vi "Stage v3.vi"() -> ()   [LabVIEW 2025]
uses:
  upper limit.ctl
  lower limit.ctl
  libximc.lvlib
panel:
  in  "Help":bool
  in  "Shift Stage Page":bool
  in  "Move to Destination Page":bool
  in  "Move Relative Page":bool
  in  "Initialize Page":bool
  in  "Tab Control":T1(tab)=enum."Shift Stage"
  out "s/n 2":u32
  out "s/n 3":u32
  out "s/n 1":u32
  in  "Controller 1":u16(ring) items=["xi-com:\\\\.\\COM4", "xi-com:\\\\.\\COM5", "xi-com:\\\\.\\COM6"]
  in  "Controller 2":u16(ring) items=["xi-com:\\\\.\\COM4", "xi-com:\\\\.\\COM5", "xi-com:\\\\.\\COM6"]
  in  "Controller 3":u16(ring) items=["xi-com:\\\\.\\COM4", "xi-com:\\\\.\\COM5", "xi-com:\\\\.\\COM6"]
  in  "Move To Destination":bool
  in  "Destination X":i32
  in  "Destination Z":i32
  in  "Destination Y":i32
  in  "Update Position":bool
  in  "Paste Positions":bool
  in  "Shift X":i32
  in  "Shift Z":i32
  in  "Shift Y":i32
  in  "Move Relative":bool
  in  "shift stage":bool
  in  "Shift Amount (Steps)":i32
  in  "Copy Positions":bool
  out "/256":i32
  out "/256":i32
  out "/256":i32
  in  "Zero":bool
  in  "Go Home":bool
  in  "Exit":bool
  out "Cursor X":dbl format="%#.2f"
  out "Cursor Z":dbl format="%#.2f"
  out "Cursor Y":dbl format="%#.2f"
  # "Controller IDs"
  # "Serial Numbers"
  # "Controller X"
  # "Controller Y"
  # "Controller Z"
  # "If serial numbers are 0, click the help button!"
  # "NOTE: Units of all positions are in steps."
  # "Stage not moving:"
  # "Check if the serial numbers are zero. If so, close this app and load the controllers in order (1, 2, then 3) in XILab. Close XILab and open this app. and controllers should load correctly."
  # "Controllers not found in XILab:"
  # "Unplug and replug USBs connecting the motors to the computer, then follow previous instructions."
  # "If you have any other questions, feel free to reach out to Erykah at erykahfoss@u.boisestate.edu"
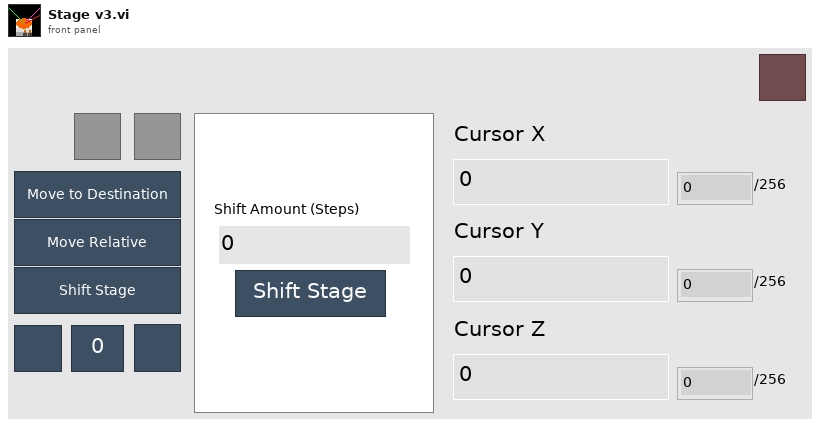
[diagram p1: front panel]
types:
  T1 = enum32{"Initialize", "Help", "Move to Destination", "Move Relative", "Shift Stage"}
  T2 = enum16{"Initialize", "Help", "Move to Destination", "Move Relative", "Shift Stage"}
  T3 = enum32{"invalid app kind", "Development System", "Run Time System", "Student Edition", "Embedded LabVIEW", "Evaluation", "Custom"}
  T4 = cluster{"Number of controllers":i32, "Controllers' names":string[], "variant":variant, "quit":bool, "IDs":i32[]}
  T5 = typedef "eventvkey.ctl" = enum16{"ASCII", "Enter", "Return", "Shift", "Ctrl", "Alt", "Cmd", "Opt", "Caps", "NumLock", "Clear", "Break", "Up", "Down", "Left", "Right", "Insert", "Delete", "Home", "End", "PageUp", "PageDown", "Escape", "Help", "Pause", "ScrollLock", "F1", "F2", "F3", "F4", "F5", "F6", "F7", "F8", "F9", "F10", "F11", "F12", "F13", "F14", "F15", "F16", "F17", "F18", "F19", "F20", "F21", "F22", "F23", "F24", "Play", "VolumeUp", "VolumeDown", "Mute", "Two Byte Char"}
  T6 = typedef "lower limit.ctl" = i32
  T7 = typedef "upper limit.ctl" = i32
  T8 = cluster{"MoveSts":u32, "MvCmdSts":u32, "PWRSts":u32, "EncSts":u32, "WindSts":u32, "CurPosition":i32, "uCurPosition":i32, "@dummy control@":i8, "@dummy control@":i8, "@dummy control@":i8, "@dummy control@":i8, "EncPosition":i64, "CurSpeed":i32, "uCurSpeed":i32, "Ipwr":i32, "Upwr":i32, "Iusb":i32, "Uusb":i32, "CurT":i32, "Flags":u32, "GPIOFlags":u32, "CmdBufFreeSpace":u32}
  T9 = cluster{"Shift Y":i32, "Shift Z":i32, "Shift X":i32}
  T10 = cluster{"Destination Y":i32, "Destination Z":i32, "Destination X":i32}
  T11 = cluster{"Shift Amount (Steps)":i32, "Shift Amount (Steps)":i32, "Shift Amount (Steps)":i32}
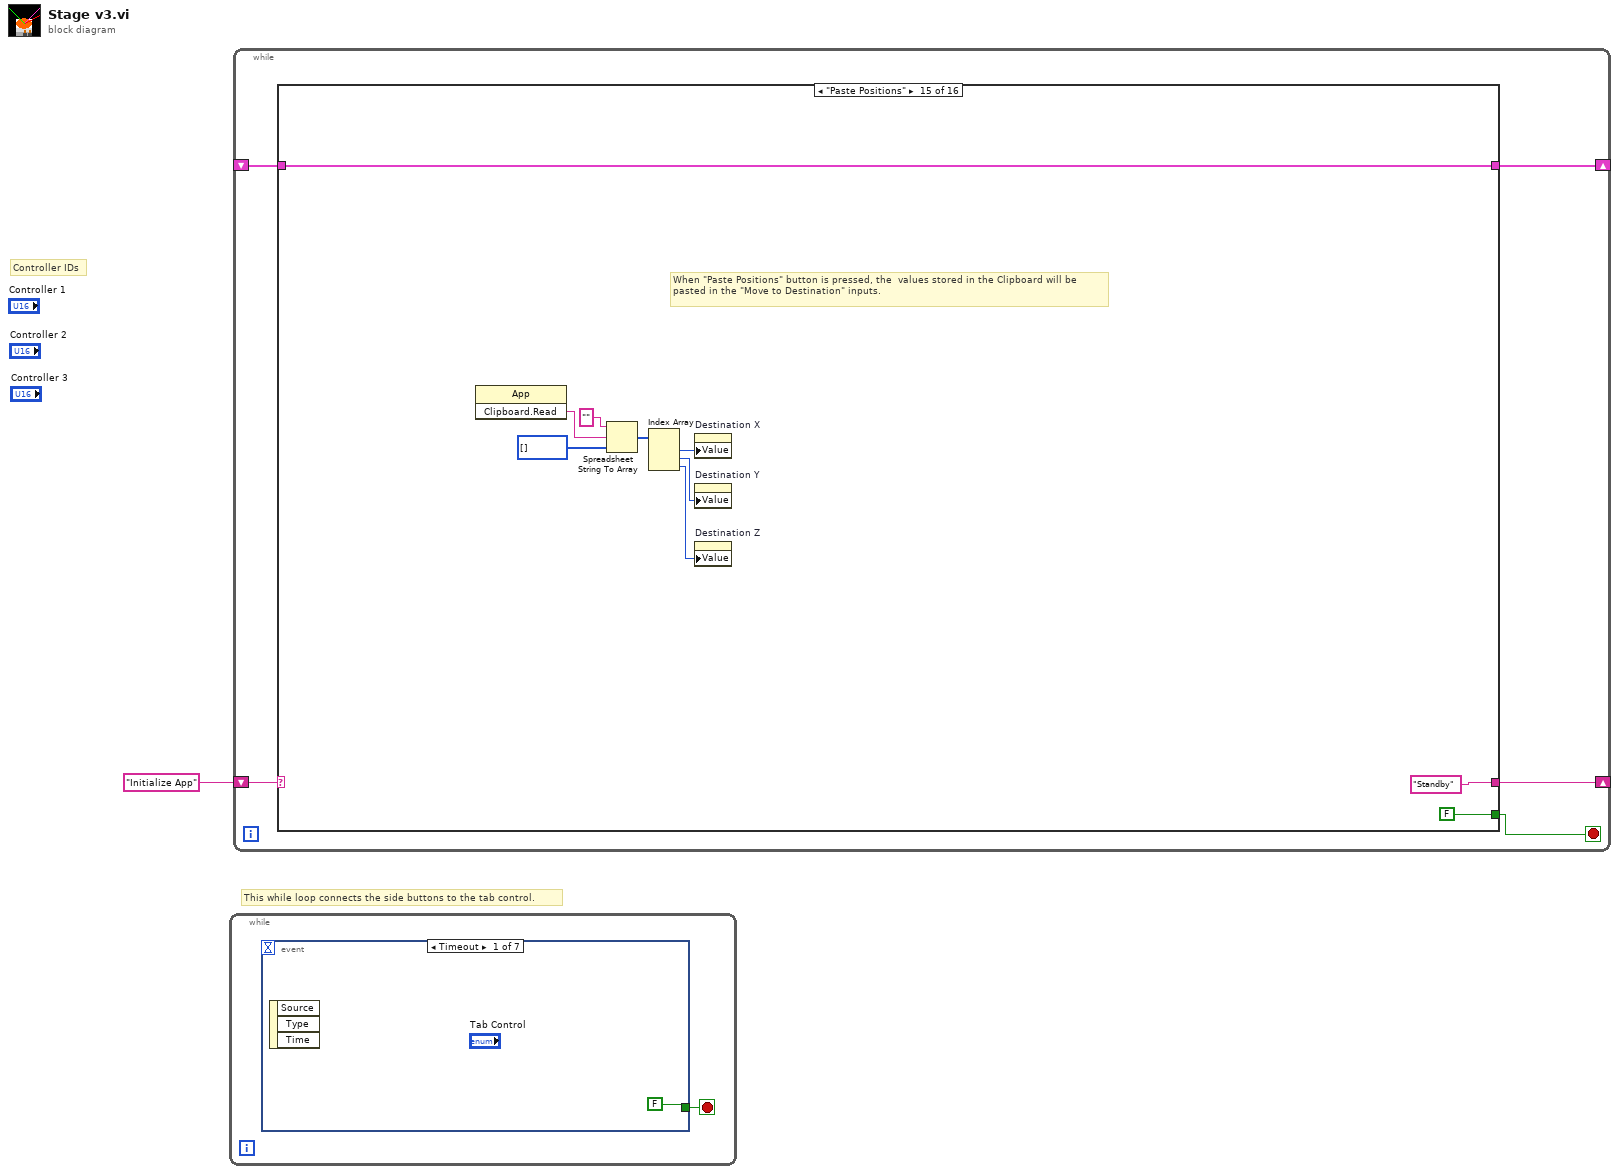
[diagram p0: block diagram]
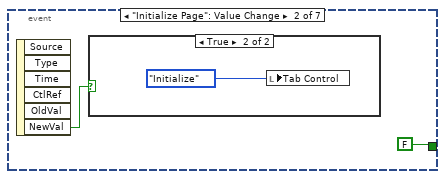
[diagram p2: hidden frame]
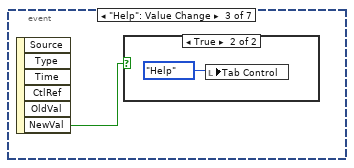
[diagram p4: hidden frame]
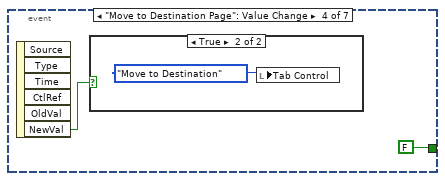
[diagram p6: hidden frame]
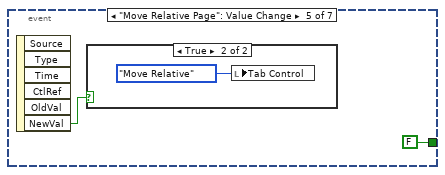
[diagram p8: hidden frame]
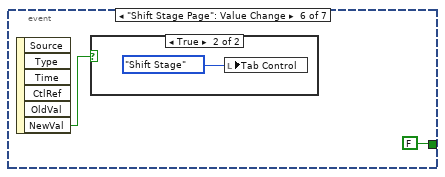
[diagram p10: hidden frame]
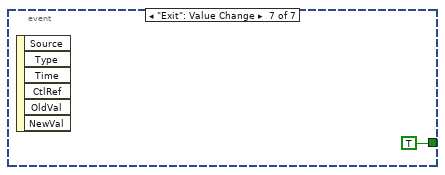
[diagram p12: hidden frame]
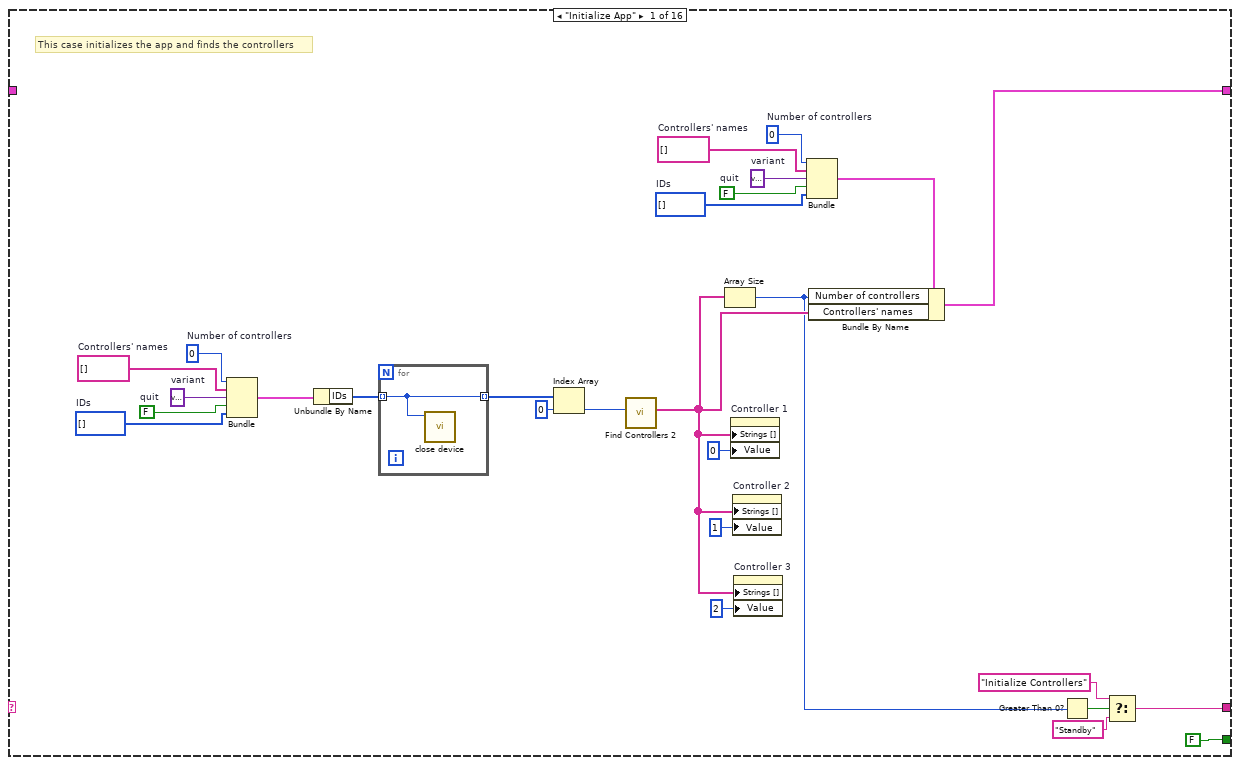
[diagram p13: hidden frame]
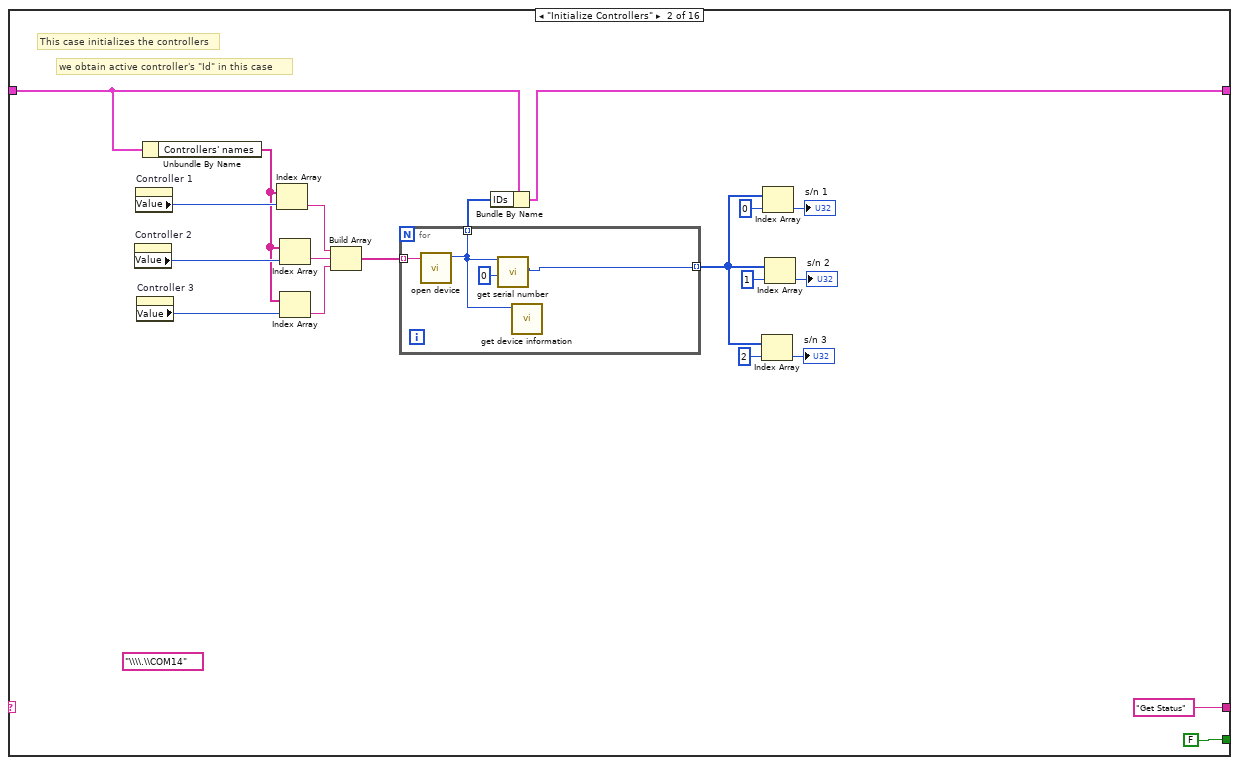
[diagram p14: hidden frame]
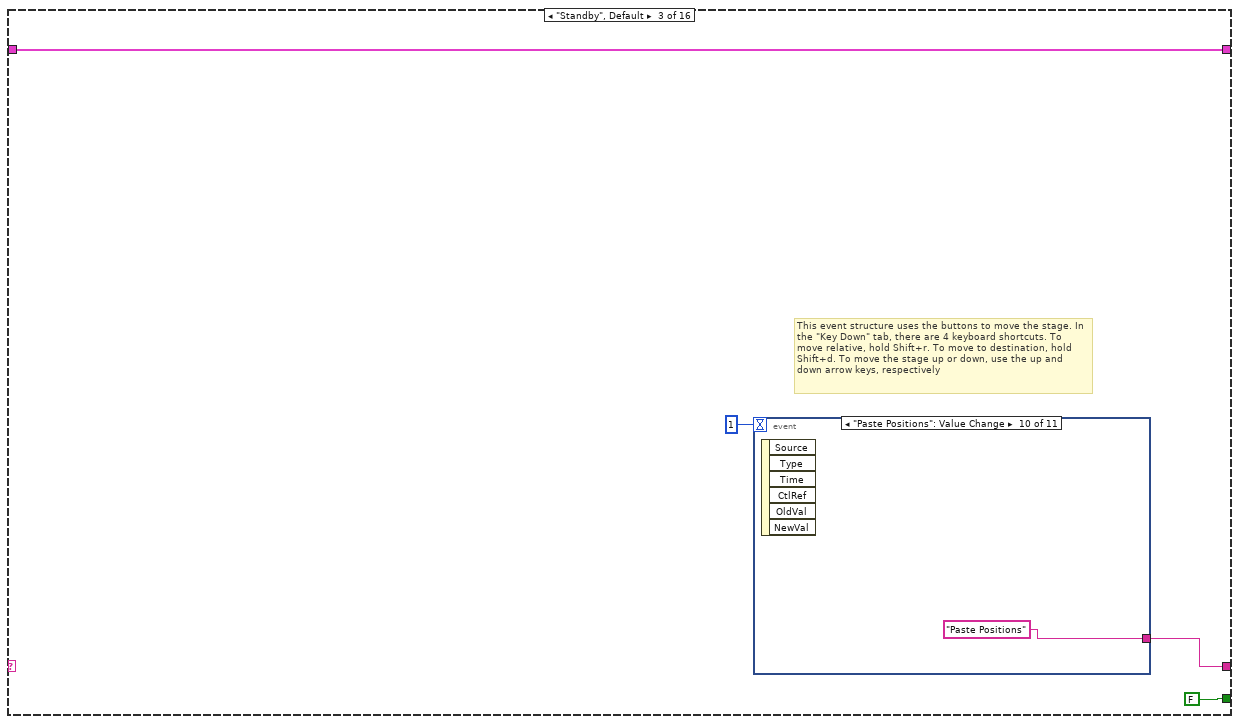
[diagram p15: hidden frame]
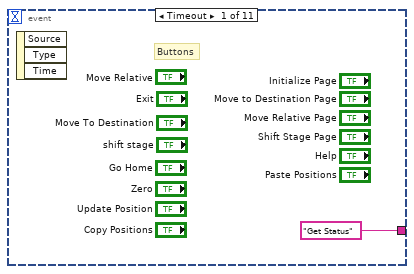
[diagram p16: hidden frame]
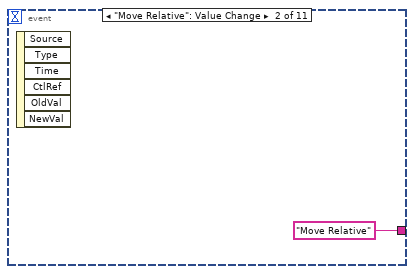
[diagram p17: hidden frame]
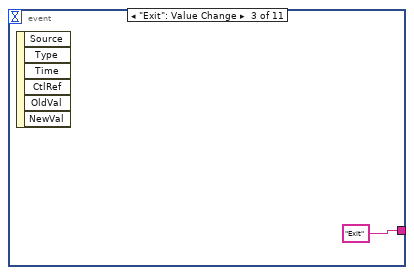
[diagram p18: hidden frame]
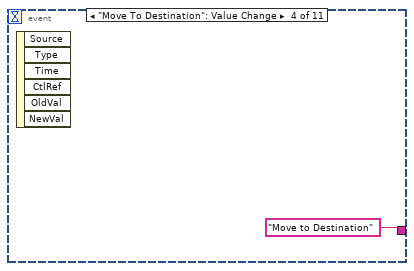
[diagram p19: hidden frame]
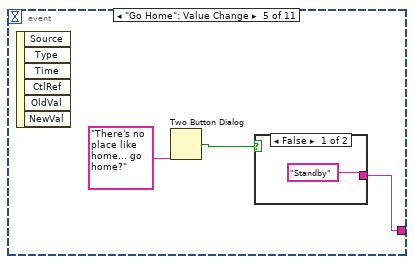
[diagram p20: hidden frame]
diagram:
  # "This while loop connects the side buttons to the tab control."
  # "Controller IDs"
  n1 = while {
    stop <- w2 stop-if-true
    n2 = event shown="[0] Timeout" {
      selector: _ -> [_ _ _ _ _ _ _]
      dyn-events: _ -> [_ _ _ _ _ _ _]
      timeout: _ -> [_ _ _ _ _ _ _]
      tunnel: [FALSE FALSE _ FALSE FALSE FALSE TRUE] -> w2
      event Timeout {
        n3 = event-data() -> ()  [unwired: 1 in, 3 out]
      }
      event "Initialize Page": Value Change {
        n4 = event-data() -> ("NewVal"=w4:bool)  [unwired: 1 in, 5 out]
        n5 = case shown="True" w4 {
          frame False {
          }
          frame True {
            n6 = local write "Tab Control"(T2."Initialize") -> ()
          }
        }
      }
      event "Help": Value Change {
        n7 = event-data() -> ("NewVal"=w7:bool)  [unwired: 1 in, 5 out]
        n8 = case shown="True" w7 {
          frame False {
          }
          frame True {
            n9 = local write "Tab Control"(T2."Help") -> ()
          }
        }
      }
      event "Move to Destination Page": Value Change {
        n10 = event-data() -> ("NewVal"=w9:bool)  [unwired: 1 in, 5 out]
        n11 = case shown="True" w9 {
          frame False {
          }
          frame True {
            n12 = local write "Tab Control"(T2."Move to Destination") -> ()
          }
        }
      }
      event "Move Relative Page": Value Change {
        n13 = event-data() -> ("NewVal"=w12:bool)  [unwired: 1 in, 5 out]
        n14 = case shown="True" w12 {
          frame False {
          }
          frame True {
            n15 = local write "Tab Control"(T2."Move Relative") -> ()
          }
        }
      }
      event "Shift Stage Page": Value Change {
        n16 = event-data() -> ("NewVal"=w15:bool)  [unwired: 1 in, 5 out]
        n17 = case shown="True" w15 {
          frame False {
          }
          frame True {
            n18 = local write "Tab Control"(T2."Shift Stage") -> ()
          }
        }
      }
      event "Exit": Value Change {
        n19 = event-data() -> ()  [unwired: 1 in, 6 out]
      }
    }
  }
  n20 = while {
    shift-right: [w22] -> _
    shift-left: _ -> [w23]
    shift-right: [w21] -> _
    shift-left: "Initialize App" -> [w20]
    stop <- w19 stop-if-true
    n21 = case shown="\"Paste Positions\"" w20 {
      tunnel: [w44 w61 w79 w118 w175 w236 w284 w341 w400 w449 w454 w459 w467 w489 w499 w507] -> w22
      tunnel: w23 -> [_ w62 w79 w118 w175 w235 w284 w341 w400 w449 w454 w459 w467 w489 w499 w507]
      tunnel: [w25 "Get Status" w77 w143 w174 w234 w283 w340 w399 "Standby" "Standby" "Standby" "Standby" "Standby" "Standby" "Standby"] -> w21
      tunnel: [FALSE ("quit") FALSE ("quit") FALSE ("quit") w130 FALSE ("quit") FALSE ("quit") FALSE FALSE FALSE FALSE FALSE FALSE FALSE FALSE FALSE TRUE ("quit")] -> w19
      frame "Initialize App" {
        w31 = i32[] []  # IDs
        w32 = FALSE  # quit
        w33 = variant  # variant
        w34 = string[] []  # Controllers' names
        w35 = 0  # Number of controllers
        w46 = i32[] []  # IDs
        w47 = FALSE  # quit
        w48 = variant  # variant
        w49 = string[] []  # Controllers' names
        w50 = 0  # Number of controllers
        # "This case initializes the app and finds the controllers"
        n22 = Bundle("Number of controllers"=w35, "Controllers' names"=w34, "variant"=w33, "quit"=w32, "IDs"=w31) -> (w30:T4)  [unwired: 1 in]
        n23 = Unbundle By Name(w30) -> ("IDs"=w37:i32[])
        n24 = for {
          tunnel: w37 -> [w51] mode=indexing
          tunnel: [w51] -> w36 mode=indexing
          n25 = call "close device.vi"("id"=w51) -> ()  [unwired: 8 in, 3 out]
        }
        n26 = Index Array(array=w36, index=0) -> (element=w42:i32)
        n27 = call "Find Controllers 2.vi"("Numeric"=w42) -> ("Names"=w38:string[])  [unwired: 9 in, 1 out]
        n28 = Array Size(array=w38) -> (size(s)=w28:i32)
        n29 = property on="Controller 1" class="Ring (strict)"("Strings []"=w38, "Value"=0) -> ()  [unwired: 2 in, 2 out]
        n30 = property on="Controller 2" class="Ring (strict)"("Strings []"=w38, "Value"=1) -> ()  [unwired: 2 in, 2 out]
        n31 = property on="Controller 3" class="Ring (strict)"("Strings []"=w38, "Value"=2 ("Controller 3")) -> ()  [unwired: 2 in, 2 out]
        n32 = Bundle("Number of controllers"=w50, "Controllers' names"=w49, "variant"=w48, "quit"=w47, "IDs"=w46) -> (w45:T4)  [unwired: 1 in]
        n33 = Bundle By Name(cluster=w45, "Number of controllers"=w28, "Controllers' names"=w38) -> (w44:T4)
        n34 = Greater Than 0?(x=w28) -> (x > 0?=w29:bool)
        n35 = Select(t="Initialize Controllers", s=w29, f="Standby") -> (s? t:f=w25:string)
      }
      frame "Initialize Controllers" {
        (unwired) "\\\\.\\COM14" ("name")
        # "we obtain active controller's \"Id\" in this case"
        # "This case initializes the controllers"
        n36 = property on="Controller 2" class="Ring (strict)"() -> ("Value"=w70:u16)  [unwired: 2 in, 2 out]
        n37 = property on="Controller 1" class="Ring (strict)"() -> ("Value"=w71:u16)  [unwired: 2 in, 2 out]
        n38 = property on="Controller 3" class="Ring (strict)"() -> ("Value"=w69:u16)  [unwired: 2 in, 2 out]
        n39 = Unbundle By Name(w62) -> ("Controllers' names"=w65:string[])
        n40 = Index Array(array=w65, index=w71) -> (element=w66:string)
        n41 = Index Array(array=w65, index=w70) -> (element=w67:string)
        n42 = Index Array(array=w65, index=w69) -> (element=w68:string)
        n43 = Build Array(w66, w67, w68) -> (w64:string[])
        n44 = for {
          tunnel: w64 -> [w75] mode=indexing
          tunnel: [w73] -> w63 mode=indexing
          tunnel: [w72] -> w54 mode=indexing
          n45 = call "open device.vi"("uri"=w75) -> ("function return"=w73:i32)  [unwired: 9 in, 1 out]
          n46 = call "get serial number.vi"("SerialNumber"=0, "id"=w73) -> ("SerialNumber out"=w72:u32)  [unwired: 7 in, 2 out]
          n47 = call "get device information.vi"("id"=w73) -> ()  [unwired: 8 in, 3 out]
        }
        n48 = Bundle By Name(cluster=w62, "IDs"=w63) -> (w61:T4)
        n49 = Index Array(array=w54, index=u32 2 ("serial")) -> (element=→"s/n 3":u32)
        n50 = Index Array(array=w54, index=u32 0 ("serial")) -> (element=→"s/n 1":u32)
        n51 = Index Array(array=w54, index=u32 1 ("serial")) -> (element=→"s/n 2":u32)
      }
      frame "Standby", Default {
        # "This event structure uses the buttons to move the stage. In the \"Key Down\" tab, there are 4 keyboard shortcuts. To move relative, hold Shift+r. To move to destination, hold Shift+d. To move the stage up or down, use the up and down arrow keys, respectively"
        n52 = event shown="[9] \"Paste Positions\": Value Change" {
          selector: _ -> [_ _ _ _ _ _ _ _ _ _ _]
          dyn-events: _ -> [_ _ _ _ _ _ _ _ _ _ _]
          timeout: 1 -> [_ _ _ _ _ _ _ _ _ _ _]
          tunnel: ["Get Status" "Move Relative" "Exit" "Move to Destination" w86 w91 "Shift Stage" "Update Position" "Copy Positions" "Paste Positions" w100] -> w77
          event Timeout {
            # "Buttons"
            n53 = event-data() -> ()  [unwired: 1 in, 3 out]
          }
          event "Move Relative": Value Change {
            n54 = event-data() -> ()  [unwired: 1 in, 6 out]
          }
          event "Exit": Value Change {
            n55 = event-data() -> ()  [unwired: 1 in, 6 out]
          }
          event "Move To Destination": Value Change {
            n56 = event-data() -> ()  [unwired: 1 in, 6 out]
          }
          event "Go Home": Value Change {
            n57 = event-data() -> ()  [unwired: 1 in, 6 out]
            n58 = Two Button Dialog(message="There's no place like home... go home?") -> (T button?=w85:bool)  [unwired: 2 in]
            n59 = case shown="False" w85 {
              tunnel: ["Standby" "Go Home"] -> w86
              frame False {
              }
              frame True {
              }
            }
          }
          event "Zero": Value Change {
            n60 = event-data() -> ()  [unwired: 1 in, 6 out]
            n61 = Two Button Dialog(message="Zero stage?") -> (T button?=w89:bool)  [unwired: 2 in]
            n62 = case shown="False" w89 {
              tunnel: ["Standby" "Zero"] -> w91
              frame False {
              }
              frame True {
              }
            }
          }
          event "shift stage": Value Change {
            n63 = event-data() -> ()  [unwired: 1 in, 6 out]
          }
          event "Update Position": Value Change {
            n64 = event-data() -> ()  [unwired: 1 in, 6 out]
          }
          event "Copy Positions": Value Change {
            n65 = event-data() -> ()  [unwired: 1 in, 6 out]
          }
          event "Paste Positions": Value Change {
            n66 = event-data() -> ()  [unwired: 1 in, 6 out]
          }
          event Key Down {
            n67 = event-data() -> ("Char"=w99:i16, "VKey"=w98:T5)  [unwired: 1 in]
            n68 = case shown="102" w99 {
              tunnel: [w101 "Move Relative" "Move to Destination" "Standby" "Standby"] -> w100
              tunnel: w98 -> [w102 _ _ _ _]
              frame 0, Default {
                n69 = case shown="\"Down\"" w102 {
                  tunnel: ["Get Status" "Shift Up" "Shift Down"] -> w101
                  frame "ASCII", Default {
                  }
                  frame "Up" {
                  }
                  frame "Down" {
                  }
                }
              }
              frame 82 {
              }
              frame 68 {
              }
              frame 102 {
                n70 = call <vilib>:"Application Directory.vi"() -> ("Application Directory"=w111:path)
                n71 = String To Path(string="f.wav") -> (path=w109:path)
                n72 = Build Path(base path=w111, name or relative path=w109) -> (appended path=w108:path)
                n73 = call <vilib>:"Play Sound File.vi"("path"=w108) -> ()  [unwired: 9 in, 2 out]
              }
              frame 108 {
                n74 = call <vilib>:"Application Directory.vi"() -> ("Application Directory"=w116:path)
                n75 = String To Path(string="l.wav") -> (path=w114:path)
                n76 = Build Path(base path=w116, name or relative path=w114) -> (appended path=w113:path)
                n77 = call <vilib>:"Play Sound File.vi"("path"=w113) -> ()  [unwired: 9 in, 2 out]
              }
            }
          }
        }
      }
      frame "Get Status" {
        w129 = T6 -600
        w131 = T7 156626
        # "y"
        # "x"
        # "z"
        # "cursor 3"
        # "cursor 2"
        # "cursor 1"
        # "lower limit"
        # "upper limit"
        # "Note: The upper limit comes from a calculation. The motor upper limit is 13 mm, and a step size is 0.083 um (https://www.standa.lt/products/catalog/motorised_positioners?item=315). The conversion is then 13 mm = 156,626 steps. Assuming that the motors are zeroed at the lowest height, the lower limit would be 0 mm = 0 steps and the upper limit would be 13 mm = 156,626 steps.\n\nMotors can't be zeroed in this LabVIEW program... this would be a good thing to include."
        # "These \"OR\" statements should check if any of the motors are at or above their upper limits or at or below thier lower limits."
        n78 = Unbundle By Name(w118) -> ("IDs"=w153:i32[])
        n79 = for {
          tunnel: [w171] -> w151 mode=indexing
          tunnel: w153 -> [w170] mode=indexing
          tunnel: [w169] -> w152 mode=indexing
          n80 = call "get status.vi"("id"=w170) -> ("status out"=w168:T8, "function return"=w169:i32)  [unwired: 8 in, 1 out]
          n81 = Unbundle By Name(w168) -> ("CurPosition"=w171:i32)
        }
        n82 = Greater Or Equal To 0?(x=w152) -> (x >= 0?=w147:bool[])
        n83 = And Array Elements(Boolean array=w147) -> ()  [unwired: 1 out]
        n84 = Index Array(array=w151, index #1=0 ("index"), index #2=1 ("index"), index #3=2 ("index")) -> (element #1=w145:i32, element #2=w138:i32, element #3=w137:i32)
        "Cursor Y" <- w145
        "Cursor Z" <- w138
        "Cursor X" <- w137
        n85 = Less?(x=w145, y=w129) -> (x < y?=w144:bool)
        n86 = Greater Or Equal?(x=w145, y=w131) -> (x >= y?=w146:bool)
        n87 = Or(x=w146, y=w144) -> (x .or. y?=w136:bool)
        n88 = Greater Or Equal?(x=w138, y=w131) -> (x >= y?=w142:bool)
        n89 = Less?(x=w138, y=w129) -> (x < y?=w141:bool)
        n90 = Or(x=w142, y=w141) -> (x .or. y?=w135:bool)
        n91 = Greater Or Equal?(x=w137, y=w131) -> (x >= y?=w140:bool)
        n92 = Less?(x=w137, y=w129) -> (x < y?=w139:bool)
        n93 = Or(x=w140, y=w139) -> (x .or. y?=w134:bool)
        n94 = Unbundle By Name(w118) -> ("IDs"=w128:i32[])
        n95 = Build Array(w136, w135, w134) -> (w133:bool[])
        n96 = Or Array Elements(Boolean array=w133) -> (logical OR=w132:bool)
        n97 = for {
          tunnel: [w157] -> w126 mode=indexing
          tunnel: w128 -> [w156] mode=indexing
          tunnel: [w155] -> w127 mode=indexing
          n98 = call "get status.vi"("id"=w156) -> ("status out"=w154:T8, "function return"=w155:i32)  [unwired: 8 in, 1 out]
          n99 = Unbundle By Name(w154) -> ("uCurPosition"=w157:i32)
        }
        n100 = case shown="False" w132 {
          tunnel: ["Standby" "Stop Motion"] -> w143
          tunnel: [FALSE w165] -> w130
          frame False {
          }
          frame True {
            # "If any of them move past the limits, the program will stop. You won't be able to use this LabVIEW program until the height is fixed in XILab."
            n101 = call <vilib>:"Application Directory.vi"() -> ("Application Directory"=w164:path)
            n102 = String To Path(string="l.wav") -> (path=w162:path)
            n103 = Build Path(base path=w164, name or relative path=w162) -> (appended path=w161:path)
            n104 = call <vilib>:"Sound File Read Simple.vi"("path"=w161) -> ("path out"=w160:path)  [unwired: 7 in, 3 out]
            n105 = call <vilib>:"Play Sound File.vi"("path"=w160) -> ()  [unwired: 9 in, 2 out]
            n106 = One Button Dialog(message="You've gone too far this time...\nPlease check the height of the stage and move it back to a normal height using XILab <3") -> (true=w165:bool)  [unwired: 1 in]
          }
        }
        n107 = Greater Or Equal To 0?(x=w127) -> (x >= 0?=w125:bool[])
        n108 = And Array Elements(Boolean array=w125) -> ()  [unwired: 1 out]
        n109 = Index Array(array=w126, index #1=0 ("index"), index #2=1 ("index"), index #3=2 ("index")) -> (element #1=→"/256":i32, element #2=→"/256":i32, element #3=→"/256":i32)
      }
      frame "Move Relative" {
        w172 = T7 156626
        w173 = -1
        # "cursor 3"
        # "cursor 2"
        # "cursor 1"
        # "lower limit"
        # "upper limit"
        n110 = Unbundle By Name(w175) -> ("IDs"=w202:i32[])
        n111 = for {
          tunnel: [w228] -> w200 mode=indexing
          tunnel: w202 -> [w227] mode=indexing
          tunnel: [w226] -> w201 mode=indexing
          n112 = call "get status.vi"("id"=w227) -> ("status out"=w225:T8, "function return"=w226:i32)  [unwired: 8 in, 1 out]
          n113 = Unbundle By Name(w225) -> ("CurPosition"=w228:i32)
        }
        n114 = Greater Or Equal To 0?(x=w201) -> (x >= 0?=w196:bool[])
        n115 = And Array Elements(Boolean array=w196) -> ()  [unwired: 1 out]
        n116 = Index Array(array=w200, index #1=0 ("index"), index #2=1 ("index"), index #3=2 ("index")) -> (element #1=w184:i32, element #2=w183:i32, element #3=w182:i32)
        n117 = Add(x="Shift Y", y=w184) -> (x+y=w181:i32)
        n118 = Add(x="Shift Z", y=w183) -> (x+y=w179:i32)
        n119 = Add(x="Shift X", y=w182) -> (x+y=w180:i32)
        n120 = Less Or Equal?(x=w181, y=w173) -> (x <= y?=w194:bool)
        n121 = Greater Or Equal?(x=w180, y=w172) -> (x >= y?=w191:bool)
        n122 = Greater Or Equal?(x=w181, y=w172) -> (x >= y?=w195:bool)
        n123 = Greater Or Equal?(x=w179, y=w172) -> (x >= y?=w193:bool)
        n124 = Less Or Equal?(x=w179, y=w173) -> (x <= y?=w192:bool)
        n125 = Less Or Equal?(x=w180, y=w173) -> (x <= y?=w190:bool)
        n126 = Or(x=w191, y=w190) -> (x .or. y?=w187:bool)
        n127 = Or(x=w193, y=w192) -> (x .or. y?=w188:bool)
        n128 = Or(x=w195, y=w194) -> (x .or. y?=w189:bool)
        n129 = Build Array(w189, w188, w187) -> (w186:bool[])
        n130 = Or Array Elements(Boolean array=w186) -> (logical OR=w185:bool)
        n131 = case shown="False" w185 {
          tunnel: ["Standby" "Stop Motion"] -> w174
          tunnel: "Shift Y" -> [w214 _]
          tunnel: "Shift Z" -> [w213 _]
          tunnel: "Shift X" -> [w212 _]
          tunnel: w175 -> [w211 w222]
          tunnel: [w209 w222] -> _
          frame False {
            n132 = Bundle("Shift Y"=w214, "Shift Z"=w213, "Shift X"=w212) -> (w210:T9)  [unwired: 1 in]
            n133 = Bundle By Name(cluster=w211, "variant"=w210) -> (w209:T4)
            n134 = Unbundle By Name(w209) -> ("IDs"=w204:i32[], "variant"=w206:variant)
            n135 = Variant To Data(type=cluster{u32, u32, u32} {0, 0, 0}, Variant=w206) -> (data=w207:cluster{u32, u32, u32})  [unwired: 1 in, 1 out]
            n136 = Cluster To Array(cluster=w207) -> (array=w208:u32[])
            n137 = for {
              tunnel: w208 -> [w216] mode=indexing
              tunnel: w204 -> [w217] mode=indexing
              n138 = call "command movr.vi"("DeltaPosition"=w216, "id"=w217) -> ()  [unwired: 8 in, 2 out]
            }
          }
          frame True {
            # "If any of them move past the limits, the motors won't move."
            n139 = call <vilib>:"Application Directory.vi"() -> ("Application Directory"=w221:path)
            n140 = String To Path(string="l.wav") -> (path=w219:path)
            n141 = Build Path(base path=w221, name or relative path=w219) -> (appended path=w218:path)
            n142 = One Button Dialog(message="You've gone too far this time...\nPlease ensure the step size does not go past the limits <3") -> ()  [unwired: 1 in, 1 out]
            n143 = call <vilib>:"Play Sound File.vi"("path"=w218) -> ()  [unwired: 9 in, 2 out]
          }
        }
      }
      frame "Move to Destination" {
        w229 = T7 156626
        w230 = -1
        # "cursor 3"
        # "cursor 2"
        # "cursor 1"
        # "lower limit"
        # "upper limit"
        n144 = Unbundle By Name(w235) -> ("IDs"=w254:i32[])
        n145 = for {
          tunnel: [w280] -> w252 mode=indexing
          tunnel: w254 -> [w279] mode=indexing
          tunnel: [w278] -> w253 mode=indexing
          n146 = call "get status.vi"("id"=w279) -> ("status out"=w277:T8, "function return"=w278:i32)  [unwired: 8 in, 1 out]
          n147 = Unbundle By Name(w277) -> ("CurPosition"=w280:i32)
        }
        n148 = Greater Or Equal To 0?(x=w253) -> (x >= 0?=w248:bool[])
        n149 = And Array Elements(Boolean array=w248) -> ()  [unwired: 1 out]
        n150 = Index Array(array=w252, index #1=0 ("index"), index #2=1 ("index"), index #3=2 ("index")) -> ()  [unwired: 3 out]
        n151 = Less Or Equal?(x="Destination Y", y=w230) -> (x <= y?=w246:bool)
        n152 = Greater Or Equal?(x="Destination X", y=w229) -> (x >= y?=w243:bool)
        n153 = Greater Or Equal?(x="Destination Y", y=w229) -> (x >= y?=w247:bool)
        n154 = Greater Or Equal?(x="Destination Z", y=w229) -> (x >= y?=w245:bool)
        n155 = Less Or Equal?(x="Destination Z", y=w230) -> (x <= y?=w244:bool)
        n156 = Less Or Equal?(x="Destination X", y=w230) -> (x <= y?=w242:bool)
        n157 = Or(x=w243, y=w242) -> (x .or. y?=w239:bool)
        n158 = Or(x=w245, y=w244) -> (x .or. y?=w240:bool)
        n159 = Or(x=w247, y=w246) -> (x .or. y?=w241:bool)
        n160 = Build Array(w241, w240, w239) -> (w238:bool[])
        n161 = Or Array Elements(Boolean array=w238) -> (logical OR=w237:bool)
        n162 = case shown="True" w237 {
          tunnel: ["Standby" "Stop Motion"] -> w234
          tunnel: "Destination Y" -> [w260 _]
          tunnel: "Destination Z" -> [w259 _]
          tunnel: "Destination X" -> [w258 _]
          tunnel: w235 -> [w257 w274]
          tunnel: [w256 w274] -> w236
          frame False {
            n163 = Bundle("Destination Y"=w260, "Destination Z"=w259, "Destination X"=w258) -> (w262:T10)  [unwired: 1 in]
            n164 = Bundle By Name(cluster=w257, "variant"=w262) -> (w256:T4)
            n165 = Unbundle By Name(w256) -> ("IDs"=w264:i32[], "variant"=w266:variant)
            n166 = Variant To Data(type=cluster{u32, u32, u32} {0, 0, 0}, Variant=w266) -> (data=w263:cluster{u32, u32, u32})  [unwired: 1 in, 1 out]
            n167 = Cluster To Array(cluster=w263) -> (array=w265:u32[])
            n168 = for {
              tunnel: w265 -> [w268] mode=indexing
              tunnel: w264 -> [w269] mode=indexing
              n169 = call "command move.vi"("Position"=w268, "id"=w269) -> ()  [unwired: 8 in, 2 out]
            }
          }
          frame True {
            # "If any of them move past the limits, the motors won't move."
            n170 = call <vilib>:"Application Directory.vi"() -> ("Application Directory"=w273:path)
            n171 = String To Path(string="l.wav") -> (path=w271:path)
            n172 = Build Path(base path=w273, name or relative path=w271) -> (appended path=w270:path)
            n173 = call <vilib>:"Play Sound File.vi"("path"=w270) -> ()  [unwired: 9 in, 2 out]
            n174 = One Button Dialog(message="You've gone too far this time...\nPlease ensure the step size does not go past the limits <3") -> ()  [unwired: 1 in, 1 out]
          }
        }
      }
      frame "Shift Stage" {
        w281 = T7 156626
        w282 = -1
        # "cursor 3"
        # "cursor 2"
        # "cursor 1"
        # "lower limit"
        # "upper limit"
        n175 = Unbundle By Name(w284) -> ("IDs"=w309:i32[])
        n176 = for {
          tunnel: [w335] -> w307 mode=indexing
          tunnel: w309 -> [w334] mode=indexing
          tunnel: [w333] -> w308 mode=indexing
          n177 = call "get status.vi"("id"=w334) -> ("status out"=w332:T8, "function return"=w333:i32)  [unwired: 8 in, 1 out]
          n178 = Unbundle By Name(w332) -> ("CurPosition"=w335:i32)
        }
        n179 = Greater Or Equal To 0?(x=w308) -> (x >= 0?=w303:bool[])
        n180 = And Array Elements(Boolean array=w303) -> ()  [unwired: 1 out]
        n181 = Index Array(array=w307, index #1=0 ("index"), index #2=1 ("index"), index #3=2 ("index")) -> (element #1=w291:i32, element #2=w290:i32, element #3=w289:i32)
        n182 = Add(x="Shift Amount (Steps)", y=w291) -> (x+y=w288:i32)
        n183 = Add(x="Shift Amount (Steps)", y=w290) -> (x+y=w286:i32)
        n184 = Add(x="Shift Amount (Steps)", y=w289) -> (x+y=w287:i32)
        n185 = Less Or Equal?(x=w288, y=w282) -> (x <= y?=w301:bool)
        n186 = Greater Or Equal?(x=w287, y=w281) -> (x >= y?=w298:bool)
        n187 = Greater Or Equal?(x=w288, y=w281) -> (x >= y?=w302:bool)
        n188 = Greater Or Equal?(x=w286, y=w281) -> (x >= y?=w300:bool)
        n189 = Less Or Equal?(x=w286, y=w282) -> (x <= y?=w299:bool)
        n190 = Less Or Equal?(x=w287, y=w282) -> (x <= y?=w297:bool)
        n191 = Or(x=w298, y=w297) -> (x .or. y?=w294:bool)
        n192 = Or(x=w300, y=w299) -> (x .or. y?=w295:bool)
        n193 = Or(x=w302, y=w301) -> (x .or. y?=w296:bool)
        n194 = Build Array(w296, w295, w294) -> (w293:bool[])
        n195 = Or Array Elements(Boolean array=w293) -> (logical OR=w292:bool)
        n196 = case shown="True" w292 {
          tunnel: ["Standby" "Stop Motion"] -> w283
          tunnel: "Shift Amount (Steps)" -> [w321 _]
          tunnel: "Shift Amount (Steps)" -> [w320 _]
          tunnel: "Shift Amount (Steps)" -> [w319 _]
          tunnel: w284 -> [w318 w329]
          tunnel: [w316 w329] -> _
          frame False {
            n197 = Bundle("Shift Amount (Steps)"=w321, "Shift Amount (Steps)"=w320, "Shift Amount (Steps)"=w319) -> (w317:T11)  [unwired: 1 in]
            n198 = Bundle By Name(cluster=w318, "variant"=w317) -> (w316:T4)
            n199 = Unbundle By Name(w316) -> ("IDs"=w311:i32[], "variant"=w313:variant)
            n200 = Variant To Data(type=cluster{u32, u32, u32} {0, 0, 0}, Variant=w313) -> (data=w314:cluster{u32, u32, u32})  [unwired: 1 in, 1 out]
            n201 = Cluster To Array(cluster=w314) -> (array=w315:u32[])
            n202 = for {
              tunnel: w315 -> [w323] mode=indexing
              tunnel: w311 -> [w324] mode=indexing
              n203 = call "command movr.vi"("DeltaPosition"=w323, "id"=w324) -> ()  [unwired: 8 in, 2 out]
            }
          }
          frame True {
            # "If any of them move past the limits, the motors won't move."
            n204 = call <vilib>:"Application Directory.vi"() -> ("Application Directory"=w328:path)
            n205 = String To Path(string="l.wav") -> (path=w326:path)
            n206 = Build Path(base path=w328, name or relative path=w326) -> (appended path=w325:path)
            n207 = call <vilib>:"Play Sound File.vi"("path"=w325) -> ()  [unwired: 9 in, 2 out]
            n208 = One Button Dialog(message="You've gone too far this time...\nPlease ensure the step size does not go past the limits <3") -> ()  [unwired: 1 in, 1 out]
          }
        }
      }
      frame "Shift Up" {
        w336 = T7 156626
        w337 = -1
        # "cursor 3"
        # "cursor 2"
        # "cursor 1"
        # "lower limit"
        # "upper limit"
        n209 = Unbundle By Name(w341) -> ("IDs"=w365:i32[])
        n210 = for {
          tunnel: [w391] -> w363 mode=indexing
          tunnel: w365 -> [w390] mode=indexing
          tunnel: [w389] -> w364 mode=indexing
          n211 = call "get status.vi"("id"=w390) -> ("status out"=w388:T8, "function return"=w389:i32)  [unwired: 8 in, 1 out]
          n212 = Unbundle By Name(w388) -> ("CurPosition"=w391:i32)
        }
        n213 = Greater Or Equal To 0?(x=w364) -> (x >= 0?=w359:bool[])
        n214 = And Array Elements(Boolean array=w359) -> ()  [unwired: 1 out]
        n215 = local read "Shift Amount (Steps)"() -> (w338:i32)
        n216 = Index Array(array=w363, index #1=0 ("index"), index #2=1 ("index"), index #3=2 ("index")) -> (element #1=w347:i32, element #2=w346:i32, element #3=w345:i32)
        n217 = Absolute Value(x=w338) -> (abs(x)=w339:i32)
        n218 = Add(x=w339, y=w347) -> (x+y=w344:i32)
        n219 = Add(x=w339, y=w346) -> (x+y=w342:i32)
        n220 = Add(x=w339, y=w345) -> (x+y=w343:i32)
        n221 = Less Or Equal?(x=w344, y=w337) -> (x <= y?=w357:bool)
        n222 = Greater Or Equal?(x=w343, y=w336) -> (x >= y?=w354:bool)
        n223 = Greater Or Equal?(x=w344, y=w336) -> (x >= y?=w358:bool)
        n224 = Greater Or Equal?(x=w342, y=w336) -> (x >= y?=w356:bool)
        n225 = Less Or Equal?(x=w342, y=w337) -> (x <= y?=w355:bool)
        n226 = Less Or Equal?(x=w343, y=w337) -> (x <= y?=w353:bool)
        n227 = Or(x=w354, y=w353) -> (x .or. y?=w350:bool)
        n228 = Or(x=w356, y=w355) -> (x .or. y?=w351:bool)
        n229 = Or(x=w358, y=w357) -> (x .or. y?=w352:bool)
        n230 = Build Array(w352, w351, w350) -> (w349:bool[])
        n231 = Or Array Elements(Boolean array=w349) -> (logical OR=w348:bool)
        n232 = case shown="True" w348 {
          tunnel: ["Standby" "Stop Motion"] -> w340
          tunnel: w339 -> [w377 _]
          tunnel: w339 -> [w376 _]
          tunnel: w339 -> [w375 _]
          tunnel: w341 -> [w374 w385]
          tunnel: [w372 w385] -> _
          frame False {
            n233 = Bundle(w377, w376, w375) -> (w373:cluster{i32, i32, i32})  [unwired: 1 in]
            n234 = Bundle By Name(cluster=w374, "variant"=w373) -> (w372:T4)
            n235 = Unbundle By Name(w372) -> ("IDs"=w367:i32[], "variant"=w369:variant)
            n236 = Variant To Data(type=cluster{u32, u32, u32} {0, 0, 0}, Variant=w369) -> (data=w370:cluster{u32, u32, u32})  [unwired: 1 in, 1 out]
            n237 = Cluster To Array(cluster=w370) -> (array=w371:u32[])
            n238 = for {
              tunnel: w371 -> [w379] mode=indexing
              tunnel: w367 -> [w380] mode=indexing
              n239 = call "command movr.vi"("DeltaPosition"=w379, "id"=w380) -> ()  [unwired: 8 in, 2 out]
            }
          }
          frame True {
            # "If any of them move past the limits, the motors won't move."
            n240 = call <vilib>:"Application Directory.vi"() -> ("Application Directory"=w384:path)
            n241 = String To Path(string="l.wav") -> (path=w382:path)
            n242 = Build Path(base path=w384, name or relative path=w382) -> (appended path=w381:path)
            n243 = call <vilib>:"Play Sound File.vi"("path"=w381) -> ()  [unwired: 9 in, 2 out]
            n244 = One Button Dialog(message="You've gone too far this time...\nPlease ensure the step size does not go past the limits <3") -> ()  [unwired: 1 in, 1 out]
          }
        }
      }
      frame "Shift Down" {
        w392 = T7 156626
        w402 = -1
        # "cursor 3"
        # "cursor 2"
        # "cursor 1"
        # "lower limit"
        # "upper limit"
        n245 = Unbundle By Name(w400) -> ("IDs"=w422:i32[])
        n246 = for {
          tunnel: [w448] -> w420 mode=indexing
          tunnel: w422 -> [w447] mode=indexing
          tunnel: [w446] -> w421 mode=indexing
          n247 = call "get status.vi"("id"=w447) -> ("status out"=w445:T8, "function return"=w446:i32)  [unwired: 8 in, 1 out]
          n248 = Unbundle By Name(w445) -> ("CurPosition"=w448:i32)
        }
        n249 = Greater Or Equal To 0?(x=w421) -> (x >= 0?=w416:bool[])
        n250 = And Array Elements(Boolean array=w416) -> ()  [unwired: 1 out]
        n251 = local read "Shift Amount (Steps)"() -> (w398:i32)
        n252 = Index Array(array=w420, index #1=0 ("index"), index #2=1 ("index"), index #3=2 ("index")) -> (element #1=w397:i32, element #2=w396:i32, element #3=w395:i32)
        n253 = Absolute Value(x=w398) -> (abs(x)=w394:i32)
        n254 = Subtract(x=w397, y=w394) -> (x-y=w404:i32)
        n255 = Subtract(x=w396, y=w394) -> (x-y=w401:i32)
        n256 = Subtract(x=w395, y=w394) -> (x-y=w403:i32)
        n257 = Less Or Equal?(x=w404, y=w402) -> (x <= y?=w414:bool)
        n258 = Greater Or Equal?(x=w403, y=w392) -> (x >= y?=w411:bool)
        n259 = Greater Or Equal?(x=w404, y=w392) -> (x >= y?=w415:bool)
        n260 = Greater Or Equal?(x=w401, y=w392) -> (x >= y?=w413:bool)
        n261 = Less Or Equal?(x=w401, y=w402) -> (x <= y?=w412:bool)
        n262 = Less Or Equal?(x=w403, y=w402) -> (x <= y?=w410:bool)
        n263 = Or(x=w411, y=w410) -> (x .or. y?=w407:bool)
        n264 = Or(x=w413, y=w412) -> (x .or. y?=w408:bool)
        n265 = Or(x=w415, y=w414) -> (x .or. y?=w409:bool)
        n266 = Negate(x=w394) -> (-x=w393:i32)
        n267 = Build Array(w409, w408, w407) -> (w406:bool[])
        n268 = Or Array Elements(Boolean array=w406) -> (logical OR=w405:bool)
        n269 = case shown="True" w405 {
          tunnel: ["Standby" "Stop Motion"] -> w399
          tunnel: w393 -> [w434 _]
          tunnel: w393 -> [w433 _]
          tunnel: w393 -> [w432 _]
          tunnel: w400 -> [w431 w442]
          tunnel: [w429 w442] -> _
          frame False {
            n270 = Bundle(w434, w433, w432) -> (w430:cluster{i32, i32, i32})  [unwired: 1 in]
            n271 = Bundle By Name(cluster=w431, "variant"=w430) -> (w429:T4)
            n272 = Unbundle By Name(w429) -> ("IDs"=w424:i32[], "variant"=w426:variant)
            n273 = Variant To Data(type=cluster{u32, u32, u32} {0, 0, 0}, Variant=w426) -> (data=w427:cluster{u32, u32, u32})  [unwired: 1 in, 1 out]
            n274 = Cluster To Array(cluster=w427) -> (array=w428:u32[])
            n275 = for {
              tunnel: w428 -> [w436] mode=indexing
              tunnel: w424 -> [w437] mode=indexing
              n276 = call "command movr.vi"("DeltaPosition"=w436, "id"=w437) -> ()  [unwired: 8 in, 2 out]
            }
          }
          frame True {
            # "If any of them move past the limits, the motors won't move."
            n277 = call <vilib>:"Application Directory.vi"() -> ("Application Directory"=w441:path)
            n278 = String To Path(string="l.wav") -> (path=w439:path)
            n279 = Build Path(base path=w441, name or relative path=w439) -> (appended path=w438:path)
            n280 = call <vilib>:"Play Sound File.vi"("path"=w438) -> ()  [unwired: 9 in, 2 out]
            n281 = One Button Dialog(message="You've gone too far this time...\nPlease ensure the step size does not go past the limits <3") -> ()  [unwired: 1 in, 1 out]
          }
        }
      }
      frame "Stop Motion" {
        n282 = Unbundle By Name(w449) -> ("IDs"=w450:i32[])
        n283 = for {
          tunnel: w450 -> [w453] mode=indexing
          n284 = call "command stop.vi"("id"=w453) -> ()  [unwired: 9 in, 2 out]
        }
      }
      frame "Go Home" {
        n285 = Unbundle By Name(w454) -> ("IDs"=w455:i32[])
        n286 = for {
          tunnel: w455 -> [w458] mode=indexing
          n287 = call "command home.vi"("id"=w458) -> ()  [unwired: 9 in, 2 out]
        }
      }
      frame "Zero" {
        n288 = Unbundle By Name(w459) -> ("IDs"=w460:i32[])
        n289 = for {
          tunnel: w460 -> [w463] mode=indexing
          n290 = call "command zero.vi"("id"=w463) -> ()  [unwired: 9 in, 2 out]
        }
      }
      frame "Update Position" {
        # "When the \"Update Position\" button is pressed, the cursor destinations in the \"Move to Destination\" tab will populate with the current cursor positions."
        n291 = Unbundle By Name(w467) -> ("IDs"=w474:i32[])
        n292 = for {
          tunnel: [w480] -> w472 mode=indexing
          tunnel: w474 -> [w479] mode=indexing
          tunnel: [w478] -> w473 mode=indexing
          n293 = call "get status.vi"("id"=w479) -> ("status out"=w477:T8, "function return"=w478:i32)  [unwired: 8 in, 1 out]
          n294 = Unbundle By Name(w477) -> ("CurPosition"=w480:i32)
        }
        n295 = Greater Or Equal To 0?(x=w473) -> (x >= 0?=w471:bool[])
        n296 = And Array Elements(Boolean array=w471) -> ()  [unwired: 1 out]
        n297 = Index Array(array=w472, index #1=0 ("index"), index #2=1 ("index"), index #3=2 ("index")) -> (element #1=w464:i32, element #2=w466:i32, element #3=w465:i32)
        n298 = local write "Destination Y"(w464) -> ()
        n299 = local write "Destination Z"(w466) -> ()
        n300 = local write "Destination X"(w465) -> ()
      }
      frame "Copy Positions" {
        # "When \"Copy Positions\" button is pressed, the current cursor values will be copied to the Clipboad. These values can then be pasted in an Excel file."
        n301 = property on="Cursor X" class="DigNum (strict)"() -> ("Value"=w488:dbl)  [unwired: 2 in, 2 out]
        n302 = property on="Cursor Y" class="DigNum (strict)"() -> ("Value"=w487:dbl)  [unwired: 2 in, 2 out]
        n303 = property on="Cursor Z" class="DigNum (strict)"() -> ("Value"=w486:dbl)  [unwired: 2 in, 2 out]
        n304 = Build Array(w488, w487, w486) -> (w485:dbl[])
        n305 = Array To Spreadsheet String(array=w485, 3:"%s" ("initial string")) -> (spreadsheet string=w484:string)  [unwired: 1 in]
        n306 = invoke class="App" method="Clipboard.Write"("Param 0"=w484) -> ()  [unwired: 3 in, 4 out]
      }
      frame "Paste Positions" {
        # "When \"Paste Positions\" button is pressed, the  values stored in the Clipboard will be pasted in the \"Move to Destination\" inputs."
        n307 = invoke class="App" method="Clipboard.Read"() -> ("Read Clipbrd"=w496:string)  [unwired: 3 in, 2 out]
        n308 = Spreadsheet String To Array(format string="", spreadsheet string=w496, array type (2D Dbl)=i32[] [] ("Array")) -> (array=w493:i32[])  [unwired: 1 in]
        n309 = Index Array(array=w493) -> (element #1=w492:i32, element #2=w491:i32, element #3=w490:i32)  [unwired: 3 in]
        n310 = property on="Destination X" class="DigNum (strict)"("Value"=w492) -> ()  [unwired: 2 in, 2 out]
        n311 = property on="Destination Y" class="DigNum (strict)"("Value"=w491) -> ()  [unwired: 2 in, 2 out]
        n312 = property on="Destination Z" class="DigNum (strict)"("Value"=w490) -> ()  [unwired: 2 in, 2 out]
      }
      frame "Exit" {
        n313 = Unbundle By Name(w507) -> ("IDs"=w509:i32[])
        n314 = for {
          tunnel: w509 -> [w510] mode=indexing
          n315 = call "close device.vi"("id"=w510) -> ()  [unwired: 8 in, 3 out]
        }
        n316 = Open Application Reference(8:errorcluster {"status"=FALSE, "code"=0, "source"=""} ("error in (no error)")) -> (0:w500:errorcluster, 3:w501:refnum<vi>)  [unwired: 3 in]
        n317 = property class="App"(reference=w501, error in=w500) -> ("App.Kind"=w504:T3)  [unwired: 2 out]
        n318 = Equal?(x=w504, y=T3."Run Time System" ("Application:Kind")) -> (x = y?=w502:bool)
        n319 = Quit LabVIEW(quit? (T)=w502) -> ()
      }
    }
  }
